vi "Stop.vi"(8 "error in (no error)":errorcluster, 10 "Message in":refnum<class "StopMessage.lvclass">, 11 "DAQMH121119OrcaFlash in":refnum<class "DAQOrcaFlash.lvclass">) -> (0 "error out":errorcluster, 3 "DAQMH121119OrcaFlash out":refnum<class "DAQOrcaFlash.lvclass">)   [LabVIEW 2012, in "DAQOrcaFlash.lvclass"]
doc: "This member function is called when the statemachine in the run.vi receives an 'stop' command. It relays the message to all observers of the component.\n\nOverride this member function in your derived class if you need additional stop functionality (but don't forget to call the parent method)."
uses:
  DAQOrcaFlash.lvclass
  <vilib>/Distrio/Murmex/Murmex/Murmex.lvclass
  imaging_mode.ctl
  <vilib>/Distrio/Murmex/StopMessage/StopMessage.lvclass
panel:
  # "This method is called when the STOP\ntrigger is sent. \n\nOverride this method when your component needs to\nrespond to this trigger. \n\nCall parent for proper implementation"
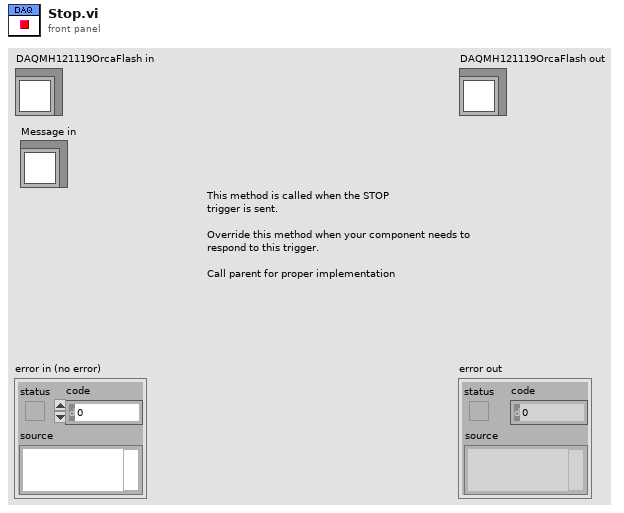
[diagram p1: front panel]
types:
  T1 = typedef "DAQOrcaFlash.lvclass/imaging_mode.ctl" = enum16{"focus mode", "single sweep"}
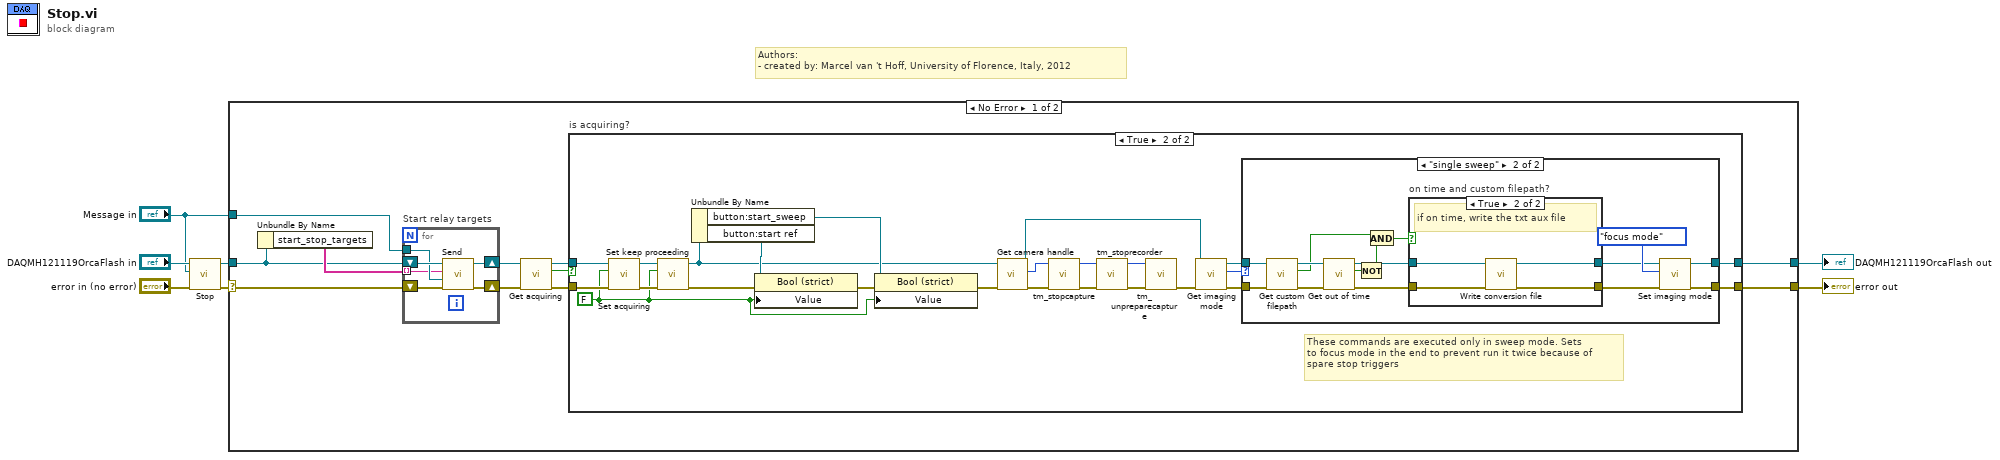
[diagram p0: block diagram]
diagram:
  # "Authors: \n- created by: Marcel van 't Hoff, University of Florence, Italy, 2012"
  n1 = call-parent "Stop.vi"("error in (no error)"="error in (no error)", "Message in"="Message in", "Murmex in"="DAQMH121119OrcaFlash in") -> ("error out"=w5:errorcluster, "Murmex out"=w2:refnum<class "DAQOrcaFlash.lvclass">)  [unwired: 7 in]
  n2 = case shown="No Error" w5 {
    selector: w5 -> [w14 w74]
    tunnel: [w9 w74] -> w4
    tunnel: [w8 w75] -> w3
    tunnel: w2 -> [w12 w75]
    tunnel: "Message in" -> [w10 _]
    frame No Error {
      n3 = Unbundle By Name(w12) -> ("start_stop_targets"=w15:string[])
      n4 = for "Start relay targets" {
        shift-right: [w24] -> w13
        shift-left: w14 -> [w23]
        tunnel: w10 -> [w21]
        tunnel: w15 -> [w20] mode=indexing
        shift-right: [w19] -> w11
        shift-left: w12 -> [w22]
        n5 = call <vilib>:"Send.vi"("error in (no error)"=w23, "Message"=w21, "recipient"=w20, "Murmex in"=w22) -> ("error out"=w24:errorcluster, "Murmex out"=w19:refnum<class "DAQOrcaFlash.lvclass">)  [unwired: 6 in]
      }
      n6 = call "Get acquiring.vi"("error in (no error)"=w13, "DAQMH121119OrcaFlash in"=w11) -> ("error out"=w17:errorcluster, "is acquiring?"=w16:bool, "DAQMH121119OrcaFlash out"=w18:refnum<class "DAQOrcaFlash.lvclass">)  [unwired: 7 in]
      n7 = case "is acquiring?" shown="True" w16 {
        tunnel: [w25 w41] -> w8
        tunnel: [w26 w42] -> w9
        tunnel: w18 -> [w25 w48]
        tunnel: w17 -> [w26 w47]
        frame False {
        }
        frame True {
          w27 = FALSE ("is acquiring?")
          # "These commands are executed only in sweep mode. Sets\nto focus mode in the end to prevent run it twice because of \nspare stop triggers"
          n8 = call "Set acquiring.vi"("error in (no error)"=w47, "is acquiring?"=w27, "DAQMH121119OrcaFlash in"=w48) -> ("error out"=w49:errorcluster, "DAQMH121119OrcaFlash out"=w29:refnum<class "DAQOrcaFlash.lvclass">)  [unwired: 7 in]
          n9 = call-dynamic "Set keep proceeding.vi"("error in (no error)"=w49, "keep proceeding?"=w27, "DAQOrcaFlash in"=w29) -> ("error out"=w30:errorcluster, "DAQOrcaFlash out"=w28:refnum<class "DAQOrcaFlash.lvclass">)  [unwired: 7 in]
          n10 = Unbundle By Name(w28) -> ("button:start_sweep"=w46:refnum<vi>, "button:start ref"=w50:refnum<vi>)
          n11 = property class="Bool (strict)"(reference=w50, error in=w30, "Value"=w27) -> (error out=w45:errorcluster)  [unwired: 1 out]
          n12 = property class="Bool (strict)"(reference=w46, error in=w45, "Value"=w27) -> (error out=w44:errorcluster)  [unwired: 1 out]
          n13 = call "Get camera handle.vi"("error in (no error)"=w44, "DAQMH121119OrcaFlash in"=w28) -> ("error out"=w34:errorcluster, "cam handle"=w33:u32, "DAQMH121119OrcaFlash out"=w39:refnum<class "DAQOrcaFlash.lvclass">)  [unwired: 7 in]
          n14 = call <userlib>:"tm_stopcapture.vi"("error in (no error)"=w34, "Handle in"=w33) -> ("error out"=w35:errorcluster, "Handle out"=w32:u32)  [unwired: 8 in]
          n15 = call <userlib>:"tm_stoprecorder.vi"("error in (no error)"=w35, "Handle in"=w32) -> ("error out"=w36:errorcluster, "Handle out"=w31:u32)  [unwired: 8 in]
          n16 = call <userlib>:"tm_unpreparecapture.vi"("error in (no error)"=w36, "Handle in"=w31) -> ("error out"=w43:errorcluster)  [unwired: 8 in, 1 out]
          n17 = call "Get imaging mode.vi"("error in (no error)"=w43, "DAQMH121119OrcaFlash in"=w39) -> ("error out"=w40:errorcluster, "imaging mode"=w37:T1, "DAQMH121119OrcaFlash out"=w38:refnum<class "DAQOrcaFlash.lvclass">)  [unwired: 7 in]
          n18 = case shown="\"single sweep\"" w37 {
            tunnel: w40 -> [w51 w60]
            tunnel: [w51 w67] -> w42
            tunnel: [w52 w66] -> w41
            tunnel: w38 -> [w52 w58]
            frame "focus mode", Default {
            }
            frame "single sweep" {
              n19 = call-dynamic "Get custom filepath.vi"("error in (no error)"=w60, "DAQOrcaFlash in"=w58) -> ("error out"=w59:errorcluster, "Custom saving path"=w54:bool, "DAQOrcaFlash out"=w57:refnum<class "DAQOrcaFlash.lvclass">)  [unwired: 7 in]
              n20 = call-dynamic "Get out of time.vi"("error in (no error)"=w59, "DAQOrcaFlash in"=w57) -> ("error out"=w61:errorcluster, "out of time?"=w56:bool, "DAQOrcaFlash out"=w62:refnum<class "DAQOrcaFlash.lvclass">)  [unwired: 7 in]
              n21 = Not(x=w56) -> (.not. x?=w55:bool)
              n22 = And(x=w54, y=w55) -> (x .and. y?=w53:bool)
              n23 = case "on time and custom filepath?" shown="True" w53 {
                tunnel: w61 -> [w68 w73]
                tunnel: [w68 w72] -> w64
                tunnel: w62 -> [w69 w71]
                tunnel: [w69 w70] -> w63
                frame False {
                  # "if out of time do nothing"
                }
                frame True {
                  # "if on time, write the txt aux file"
                  n24 = call-dynamic "Write conversion file.vi"("error in (no error)"=w73, "DAQOrcaFlash in"=w71) -> ("error out"=w72:errorcluster, "DAQOrcaFlash out"=w70:refnum<class "DAQOrcaFlash.lvclass">)  [unwired: 8 in]
                }
              }
              n25 = call "Set imaging mode.vi"("error in (no error)"=w64, "imaging mode"=imaging_mode."focus mode", "DAQMH121119OrcaFlash in"=w63) -> ("error out"=w67:errorcluster, "DAQMH121119OrcaFlash out"=w66:refnum<class "DAQOrcaFlash.lvclass">)  [unwired: 7 in]
            }
          }
        }
      }
    }
    frame Error {
    }
  }
  "error out" <- w4
  "DAQMH121119OrcaFlash out" <- w3
